vi "Template.vi"() -> ()   [LabVIEW 2019, in "Template.lvlib"]
doc: "This template is for the Queued Message Handler design pattern.\n\nThe Event Handling Loop generates messages based on user interface actions.\n\nThe Message Handling Loop processes messages generated by the Event Handling Loop, or by other messages. The messages are string values, so new messages can be added easily to the Message Cases case structure in the Message Handling Loop. Each message cluster can also provide an optional value for Message Data, which is a variant that can be converted to whatever message-specific data is required.a"
uses:
  Template.lvlib
  Data.ctl
  Message Queue/State Name.ctl
  Support/Message Queue/State Name.ctl
  <vilib>/event_ctls.llb/usereventprio.ctl
  0c61461a-fa07-4497-8c8c-8d3ef654e9c8.vi
  bad579f2-958a-4e04-a1a5-1778729f7708.vi
  681f6a39-68c9-4eb8-ab39-fd2fc03f9966.vi
  <vilib>/Utility/error.llb/Clear Errors.vi
  Message Queue/Enqueue (Single).vi
  <vilib>/Utility/error.llb/Error Cluster From Error Code.vi
  Message Queue/Enqueue (Array).vi
  Support/Message Queue/Reference Queue.vi
  <vilib>/ErrorRing/Error Ring.xnode
  Support/Message Queue/Message Queue.lvlib
panel:
  out "Headline":string
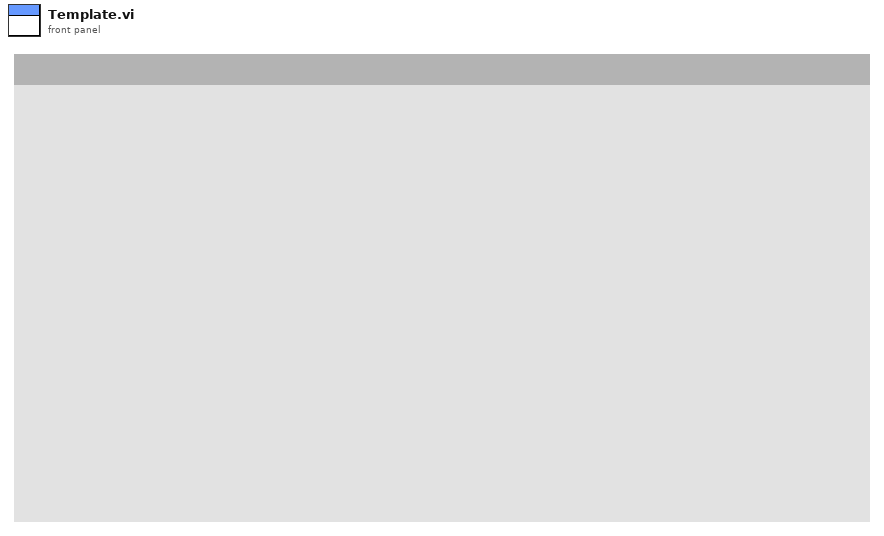
[diagram p1: front panel]
types:
  T1 = typedef "Template.lvlib/State Name.ctl" = enum16{"Default", "Initialize", "Re-Initialize", "Initialize Data", "Initialize Panel", "[Event Structure] Update Data", "Error", "Exit"}
  T2 = typedef "Template.lvlib/Data.ctl" = cluster{"Exit":bool, "States":T1}
  T3 = typedef "Message Queue Ref.ctl" = refnum<queue>
  T4 = typedef "Message Queue.lvlib/State Name.ctl" = enum16{"Default", "Initialize", "Initialize Data", "Initialize Modules", "Initialize Panel", "Close FP", "Open FP", "Initialize Menu", "Mode", "Update Subpanel", "Error", "Open Help", "About", "Open WebResources", "Exit"}
  T5 = typedef "usereventprio.ctl" = enum32{"high priority", "normal priority"}
  T6 = cluster{"Call Chain":string[], "Custom State Name":string, "timed out?":bool}
  T7 = enum16{"Left Button", "Center Button", "Right Button", "Window Close"}
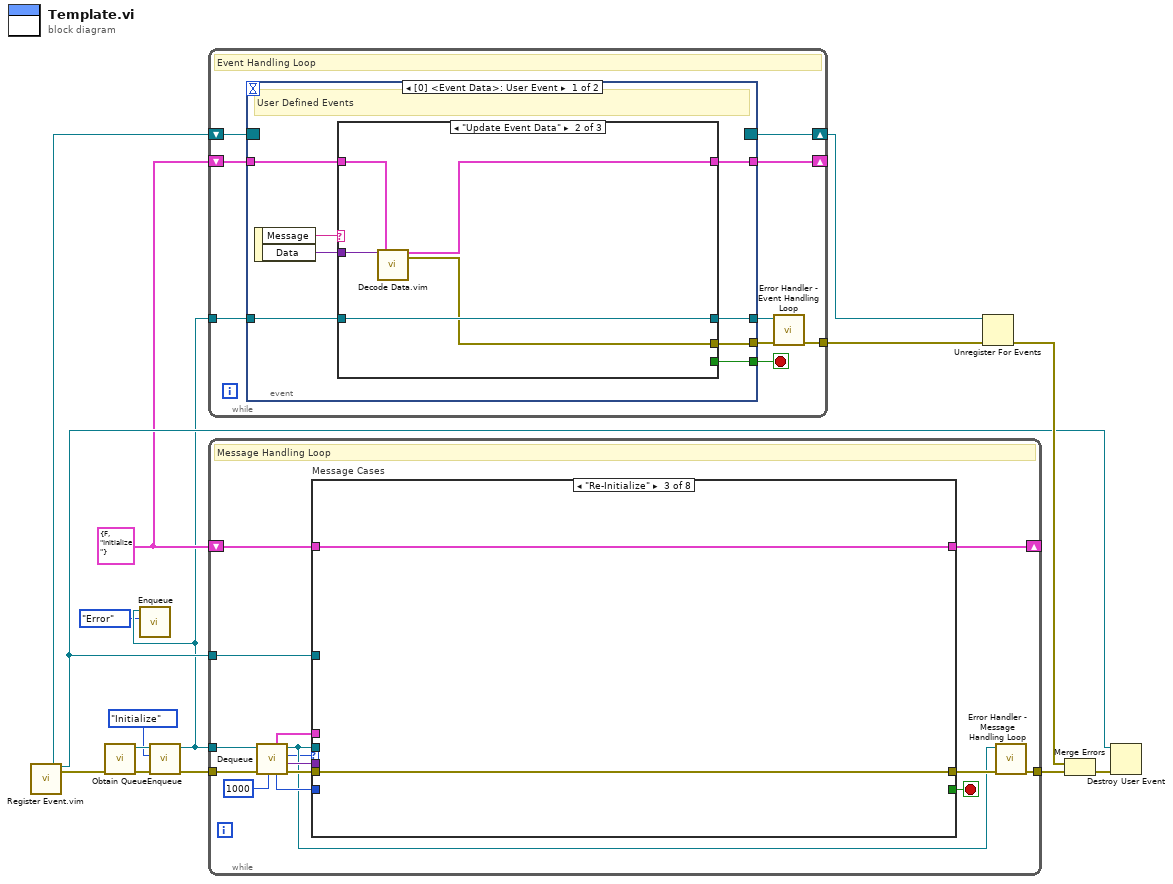
[diagram p0: block diagram]
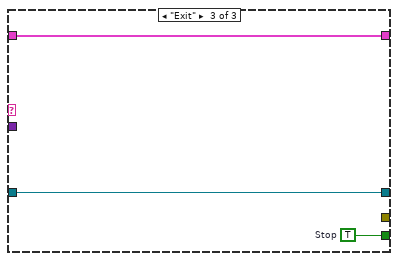
[diagram p3: hidden frame]
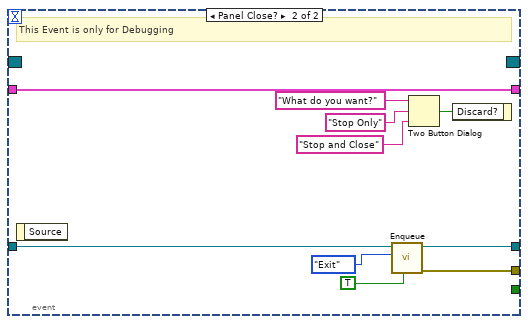
[diagram p4: hidden frame]
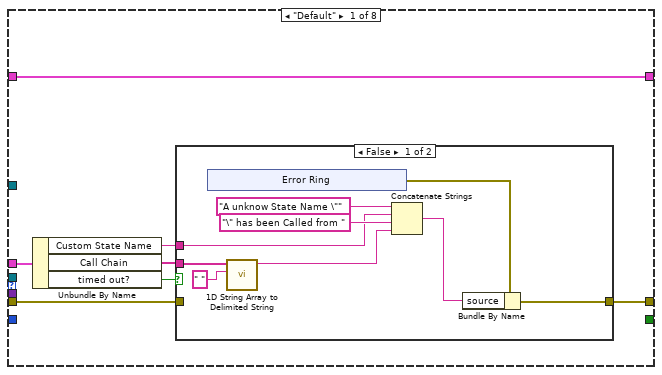
[diagram p5: hidden frame]
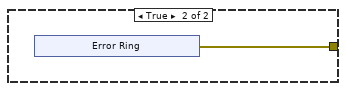
[diagram p6: hidden frame]
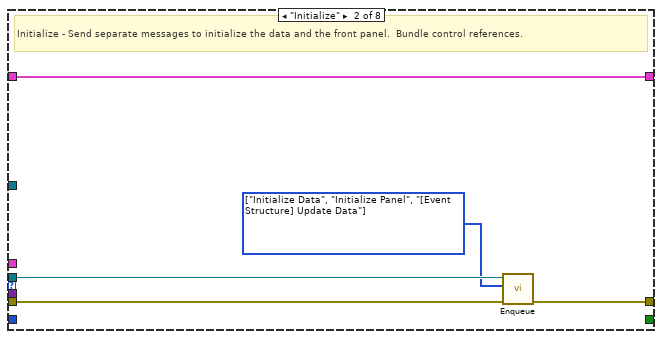
[diagram p7: hidden frame]
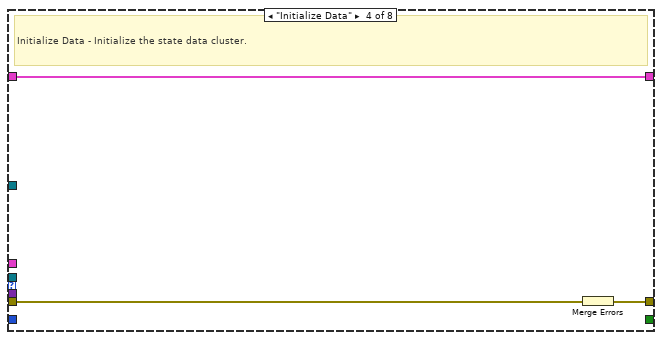
[diagram p8: hidden frame]
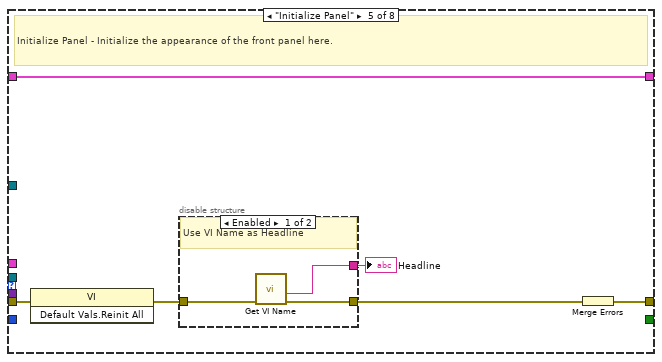
[diagram p9: hidden frame]
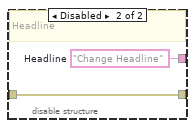
[diagram p10: hidden frame]
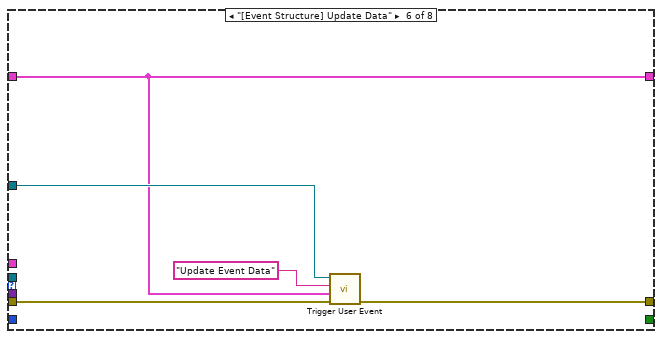
[diagram p11: hidden frame]
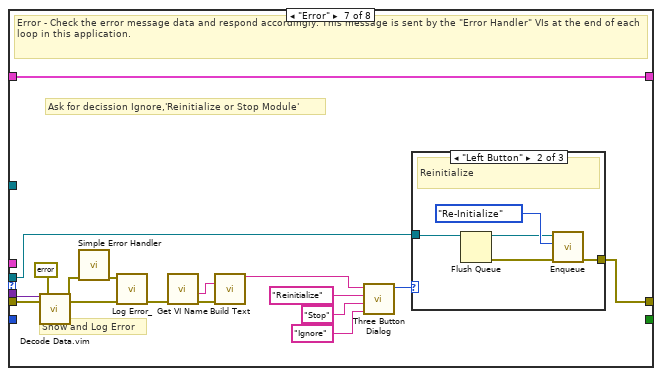
[diagram p12: hidden frame]
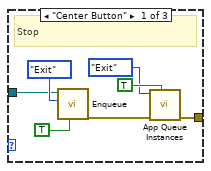
[diagram p13: hidden frame]
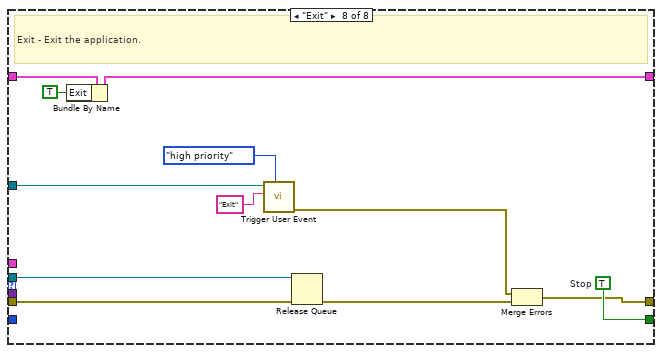
[diagram p15: hidden frame]
diagram:
  w4 = T2 {"Exit"=FALSE, "States"=enum."Initialize"} ("Data")
  n1 = call "Register Event.vim"() -> ("Registration"=w3:refnum<event-registration>, "user event out"=w6:refnum<user-event>, "error out"=w7:errorcluster)  [unwired: 17 in]
  n2 = call "Obtain Queue.vi"("error in (no error)"=w7) -> ("error out"=w11:errorcluster, "Message out"=w12:T3)  [unwired: 9 in]
  n3 = call-poly "Enqueue.vi"("error in (no error)"=w11, "States"=State_Name."Initialize", "Message Queue"=w12) -> ("error out"=w10:errorcluster, "Message Queue dub"=w2:T3)  [unwired: 7 in]
  n4 = call-poly "Enqueue.vi"("States"=State_Name."Error", "Message Queue"=w2) -> ()  [unwired: 8 in, 2 out]
  n5 = while {
    tunnel: w2 -> [w24]
    shift-right: [w16] -> w9
    shift-left: w3 -> [w17]
    tunnel: [w21] -> w13
    shift-right: [w18] -> _
    shift-left: w4 -> [w19]
    stop <- w23 stop-if-true
    # "Event Handling Loop"
    n6 = event shown="[0] <Event Data>: User Event" {
      selector: w17 -> [_ _]
      dyn-events: [_ _] -> w16
      timeout: _ -> [_ _]
      tunnel: [w32 _] -> w23
      tunnel: w24 -> [w29 w45]
      tunnel: [w31 w46] -> w20
      tunnel: [w30 w47] -> w22
      tunnel: w19 -> [w27 w43]
      tunnel: [w28 w43] -> w18
      event User Event {
        # "User Defined Events"
        n7 = event-data() -> ("Message"=w26:string, "Data"=w25:variant)  [unwired: 1 in]
        n8 = case shown="\"Update Event Data\"" w26 {
          tunnel: [_ _ w42] -> w32
          tunnel: [_ w35 _] -> w31
          tunnel: w25 -> [_ w39 _]
          tunnel: [w34 w36 w41] -> w30
          tunnel: w29 -> [w34 w36 w41]
          tunnel: [w33 w37 w40] -> w28
          tunnel: w27 -> [w33 w38 w40]
          frame Default {
          }
          frame "Update Event Data" {
            n9 = call "Decode Data.vim"("Data"=w39, "Type/Default value"=w38) -> ("Data out"=w37:T2, "error out"=w35:errorcluster)  [unwired: 16 in]
          }
          frame "Exit" {
            w42 = TRUE  # Stop
          }
        }
      }
      event Panel Close? {
        # "This Event is only for Debugging"
        n10 = event-data() -> ()  [unwired: 1 in, 1 out]
        n11 = call-poly "Enqueue.vi"("Priority Message? Array"=TRUE ("Priority Message? (F)"), "States"=State_Name."Exit" ("Array"), "Message Queue"=w45) -> ("error out"=w46:errorcluster, "Message Queue dub"=w47:T3)  [unwired: 7 in]
        n12 = Two Button Dialog(message="What do you want?", 1:"Stop and Close" ("F button name (\"Cancel\")"), 2:"Stop Only" ("T button name (\"OK\")")) -> (T button?=w49:bool)
        n13 = event-data("Discard?"=w49) -> ()  [unwired: 1 in, 1 out]
      }
    }
    n14 = call "Error Handler - Event Handling Loop.vi"("error in (no error)"=w20, "Message Queue"=w22) -> ("dup error in"=w21:errorcluster)  [unwired: 8 in, 1 out]
  }
  n15 = while {
    tunnel: w2 -> [w61]
    tunnel: w10 -> [w64]
    tunnel: [w60] -> w15
    shift-right: [w56] -> _
    shift-left: w4 -> [w66]
    tunnel: w6 -> [w55]
    stop <- w65 stop-if-true
    # "Message Handling Loop"
    n16 = call "Dequeue.vi"("timeout in ms (-1)"=1000, "error in (no error)"=w64, "Message Queue"=w61) -> ("error out"=w63:errorcluster, "Message Data"=w62:variant, "State"=w57:T1, "Message Queue dub"=w58:T3, "# elements in queue"=w67:i32, "Caller Info"=w53:T6)  [unwired: 3 in]
    n17 = case "Message Cases" shown="\"Re-Initialize\"" w57 {
      tunnel: w58 -> [_ w97 _ _ _ _ w122 w160]
      tunnel: w63 -> [w73 w94 w100 w101 w107 w119 w131 w156]
      tunnel: [w72 w98 w100 w103 w109 w118 w121 w157] -> w59
      tunnel: w66 -> [w74 w96 w99 w102 w108 w116 w136 w155]
      tunnel: [_ _ _ _ _ _ _ w159] -> w65
      tunnel: w62 -> [_ _ _ _ _ _ w128 _]
      tunnel: [w74 w96 w99 w102 w108 w116 w136 w153] -> w56
      tunnel: w55 -> [_ _ _ _ _ w117 _ w152]
      tunnel: w67 -> [_ _ _ _ _ _ _ _]
      tunnel: w53 -> [w71 _ _ _ _ _ _ _]
      frame "Default" {
        n18 = Unbundle By Name(w71) -> ("Custom State Name"=w69:string, "Call Chain"=w70:string[], "timed out?"=w68:bool)
        n19 = case shown="False" w68 {
          tunnel: w73 -> [_ _]
          tunnel: [w81 w88] -> w72
          tunnel: w70 -> [w76 _]
          tunnel: w69 -> [w75 _]
          frame False {
            n20 = xnode "Error Ring"() -> ("error out"=w83:errorcluster)
            n21 = call <vilib>:"1D String Array to Delimited String.vi"("delimiter"=" ", "string array"=w76) -> ("delimited string"=w77:string)  [unwired: 9 in]
            n22 = Concatenate Strings("A unknow State Name \"" ("source"), w75, "\" has been Called from " ("string"), w77) -> (w79:string)
            n23 = Bundle By Name(cluster=w83, "source"=w79) -> (w81:errorcluster)
          }
          frame True {
            n24 = xnode "Error Ring"() -> ("error out"=w88:errorcluster)
          }
        }
      }
      frame "Initialize" {
        w95 = T1[] [enum."Initialize Data", enum."Initialize Panel", enum."[Event Structure] Update Data"] items=["Default", "Initialize", "Re-Initialize", "Initialize Data", "Initialize Panel", "[Event Structure] Update Data", "Error", "Exit"] ("Array")
        # "Initialize - Send separate messages to initialize the data and the front panel.  Bundle control references."
        n25 = call-poly "Enqueue.vi"("error in (no error)"=w94, "States"=w95, "Message Queue"=w97) -> ("error out"=w98:errorcluster)  [unwired: 7 in, 1 out]
      }
      frame "Re-Initialize" {
      }
      frame "Initialize Data" {
        # "Initialize Data - Initialize the state data cluster."
        n26 = Merge Errors(w101) -> (w103:errorcluster)
      }
      frame "Initialize Panel" {
        # "Initialize Panel - Initialize the appearance of the front panel here."
        n27 = invoke class="VI" method="Default Vals.Reinit All"(error in=w107) -> (error out=w106:errorcluster)  [unwired: 2 in, 2 out]
        n28 = disable-structure shown="Enabled" {
          disable-tunnel: w106 -> [w112 w113]
          disable-tunnel: [w111 w113] -> w104
          disable-tunnel: [w110 w114] -> w105
          frame Enabled {
            # "Use VI Name as Headline"
            n29 = call "Get VI Name.vi"("error in (no error)"=w112) -> ("error out"=w111:errorcluster, "VI Name without extension"=w110:string)  [unwired: 8 in, 1 out]
          }
          frame Disabled {
            w114 = "Change Headline"  # Headline
            # "Headline"
          }
        }
        "Headline" <- w105
        n30 = Merge Errors(w104) -> (w109:errorcluster)
      }
      frame "[Event Structure] Update Data" {
        n31 = call "Trigger User Event.vi"("error in (no error)"=w119, "Message Data"=w116, "Message"="Update Event Data", "user event in"=w117) -> ("error out"=w118:errorcluster)  [unwired: 6 in, 1 out]
      }
      frame "Error" {
        # "Ask for decission Ignore,'Reinitialize or Stop Module'"
        # "Show and Log Error"
        # "Error - Check the error message data and respond accordingly. This message is sent by the \"Error Handler\" VIs at the end of each loop in this application."
        n32 = call "Decode Data.vim"("Data"=w128, "error in"=w131, "Type/Default value"=errorcluster {"status"=FALSE, "code"=0, "source"=""} ("error constant")) -> ("Data out"=w129:errorcluster, "error out"=w127:errorcluster)  [unwired: 15 in]
        n33 = call <vilib>:"Simple Error Handler.vi"("error in (no error)"=w129) -> ("error out"=w135:errorcluster)  [unwired: 4 in, 4 out]
        n34 = call "Log Error_.vi"("error in"=w127, "Error log to file"=w135) -> ("error out"=w134:errorcluster)  [unwired: 9 in]
        n35 = call "Get VI Name.vi"("error in (no error)"=w134) -> ("error out"=w132:errorcluster, "VI Name without extension"=w133:string)  [unwired: 8 in, 1 out]
        n36 = call "Build Text"("ModuleName"=w133, "error in (no error)"=w132) -> ("Result"=w120:string)  [unwired: 12 in, 1 out]
        n37 = call <vilib>:"Three Button Dialog.vi"("Right Button Text (\"Cancel\")"="Ignore" ("Right Button Text (\"Cancel\")"), "Center Button Text (\"No\")"="Stop" ("Center Button Text (\"No\")"), "Left Button Text (\"Yes\")"="Reinitialize" ("Left Button Text (\"Yes\")"), "message"=w120) -> ("Which Button?"=w126:T7)  [unwired: 7 in]
        n38 = case shown="\"Left Button\"" w126 {
          tunnel: w122 -> [w138 w144 _]
          tunnel: [w137 w145 _] -> w121
          frame "Center Button" {
            # "Stop"
            n39 = call-poly "Enqueue.vi"("Priority Message? Array"=TRUE ("Priority Message? (F)"), "States"=State_Name."Exit" ("Array"), "Message Queue"=w138) -> ("error out"=w143:errorcluster)  [unwired: 7 in, 1 out]
            n40 = call-poly "App Queue Instances.vi"("Priority Message? (F)"=TRUE, "error in (no error)"=w143, "Tasks"=State_Name."Exit") -> ("error out"=w137:errorcluster)  [unwired: 8 in]
          }
          frame "Left Button" {
            # "Reinitialize"
            n41 = Flush Queue(queue=w144) -> (queue out=w146:T3, error out=w147:errorcluster)  [unwired: 1 in, 1 out]
            n42 = call-poly "Enqueue.vi"("error in (no error)"=w147, "States"=State_Name."Re-Initialize" ("Array"), "Message Queue"=w146) -> ("error out"=w145:errorcluster)  [unwired: 7 in, 1 out]
          }
          frame "Right Button", "Window Close" {
          }
        }
      }
      frame "Exit" {
        w159 = TRUE  # Stop
        # "Exit - Exit the application."
        n43 = Bundle By Name(cluster=w155, "Exit"=TRUE) -> (w153:T2)
        n44 = call "Trigger User Event.vi"("priority (normal)"=usereventprio."high priority", "Message"="Exit", "user event in"=w152) -> ("error out"=w151:errorcluster)  [unwired: 7 in, 1 out]
        n45 = Release Queue(queue=w160, error in (no error)=w156) -> (error out=w158:errorcluster)  [unwired: 1 in, 2 out]
        n46 = Merge Errors(w151, w158) -> (w157:errorcluster)
      }
    }
    n47 = call "Error Handler - Message Handling Loop.vi"("error in (no error)"=w59, "Message Queue"=w58) -> ("dup error in"=w60:errorcluster)  [unwired: 8 in, 1 out]
  }
  n48 = Unregister For Events(event registration refnum=w9, error in=w13) -> (error out=w14:errorcluster)
  n49 = Merge Errors(w14, w15) -> (w8:errorcluster)
  n50 = Destroy User Event(user event=w6, error in=w8) -> ()  [unwired: 1 out]
